vi "Open.vi"(6 "timeout":i32=3, 8 "error in (no error)":errorcluster, 10 "nbaud":i32=115200, 11 "Serial Port":string) -> (0 "error out":errorcluster, 3 "hDevice":i32, 5 "Connected?":bool)   [LabVIEW 2011, in "Thorlabs_MDT69xB.lvlib"]
doc: "Open com port."
uses:
  <instrlib>/Thorlabs_MDT69xB/Thorlabs_MDT69xB.lvlib
  <instrlib>/Thorlabs_MDT69xB/Data/MDT_COMMAND_LIB_win32.dll
  <instrlib>/Thorlabs_MDT69xB/Data/MDT_COMMAND_LIB_x64.dll
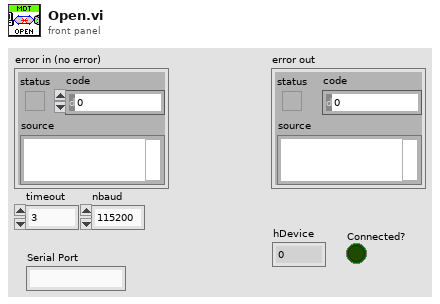
[diagram p1: front panel]
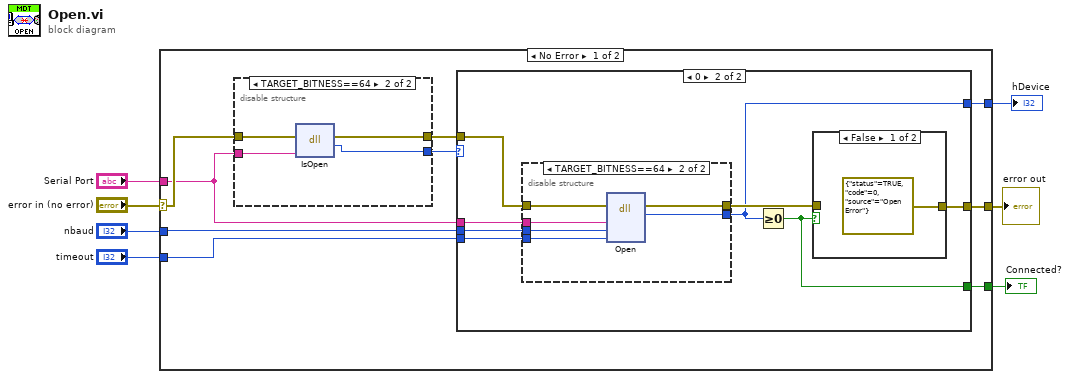
[diagram p0: block diagram]
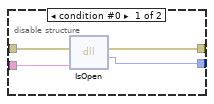
[diagram p2: hidden frame]
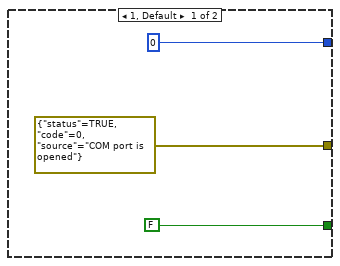
[diagram p3: hidden frame]
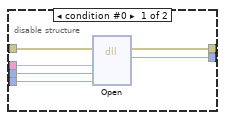
[diagram p4: hidden frame]
diagram:
  n1 = case shown="No Error" "error in (no error)" {
    selector: "error in (no error)" -> [w11 w50]
    tunnel: [w16 w50] -> w6
    tunnel: "timeout" -> [w14 _]
    tunnel: "nbaud" -> [w15 _]
    tunnel: "Serial Port" -> [w8 _]
    tunnel: [w13 _] -> w2
    tunnel: [w12 _] -> w1
    frame No Error {
      n2 = disable-structure shown="TARGET_BITNESS==64" {
        disable-tunnel: w8 -> [w20 w24]
        disable-tunnel: w11 -> [w19 w23]
        disable-tunnel: [w18 w22] -> w10
        disable-tunnel: [w17 w21] -> w9
        frame condition #0 {
          n3 = dll-call lib="C:/Program Files (x86)/National Instruments/LabVIEW 2011/instr.lib/Thorlabs_MDT69xB/Data/MDT_COMMAND_LIB_win32.dll" fn="IsOpen"(error in=w19, "Serial Number"=w20) -> (error out=w18:errorcluster, "return type"=w17:i32)  [unwired: 3 in, 1 out]
        }
        frame condition #1 (active) {
          n4 = dll-call lib="C:/Program Files/National Instruments/LabVIEW 2011/instr.lib/Thorlabs_MDT69xB/Data/MDT_COMMAND_LIB_x64.dll" fn="IsOpen"(error in=w23, "Serial Number"=w24) -> (error out=w22:errorcluster, "return type"=w21:i32)  [unwired: 3 in, 1 out]
        }
      }
      n5 = case shown="0" w9 {
        tunnel: [errorcluster {"status"=TRUE, "code"=0, "source"="COM port is opened"} ("error out") w35] -> w16
        tunnel: w15 -> [_ w34]
        tunnel: w14 -> [_ w33]
        tunnel: [0 ("return type") w31] -> w13
        tunnel: [FALSE w30] -> w12
        tunnel: w8 -> [_ w29]
        tunnel: w10 -> [_ w28]
        frame 1, Default {
        }
        frame 0 {
          n6 = disable-structure shown="TARGET_BITNESS==64" {
            disable-tunnel: w34 -> [w41 w47]
            disable-tunnel: w33 -> [w40 w46]
            disable-tunnel: [w39 w45] -> w32
            disable-tunnel: [w38 w44] -> w31
            disable-tunnel: w29 -> [w37 w43]
            disable-tunnel: w28 -> [w36 w42]
            frame condition #0 {
              n7 = dll-call lib="C:/Program Files (x86)/National Instruments/LabVIEW 2011/instr.lib/Thorlabs_MDT69xB/Data/MDT_COMMAND_LIB_win32.dll" fn="Open"(error in=w36, "Serial Number"=w37, "nbaud"=w41, "timeout"=w40) -> (error out=w39:errorcluster, "return type"=w38:i32)  [unwired: 5 in, 1 out]
            }
            frame condition #1 (active) {
              n8 = dll-call lib="C:/Program Files/National Instruments/LabVIEW 2011/instr.lib/Thorlabs_MDT69xB/Data/MDT_COMMAND_LIB_x64.dll" fn="Open"(error in=w42, "Serial Number"=w43, "nbaud"=w47, "timeout"=w46) -> (error out=w45:errorcluster, "return type"=w44:i32)  [unwired: 5 in, 1 out]
            }
          }
          n9 = Greater Or Equal To 0?(x=w31) -> (x >= 0?=w30:bool)
          n10 = case shown="False" w30 {
            tunnel: w32 -> [_ w49]
            tunnel: [errorcluster {"status"=TRUE, "code"=0, "source"="Open Error"} ("error out") w49] -> w35
            frame False {
            }
            frame True {
            }
          }
        }
      }
    }
    frame Error {
    }
  }
  "error out" <- w6
  "hDevice" <- w2
  "Connected?" <- w1
